vi "Output on.vi"(8 "error in (no error)":errorcluster, 10 "Output On":bool, 11 "Power Supply in":refnum<class "Power Supply.lvclass">) -> (0 "error out":errorcluster, 3 "Power Supply out":refnum<class "Power Supply.lvclass">)   [LabVIEW 2020, in "Power Supply.lvclass"]
uses:
  Power Supply.lvclass
  Power Supply.lvclass/Power Supply.ctl
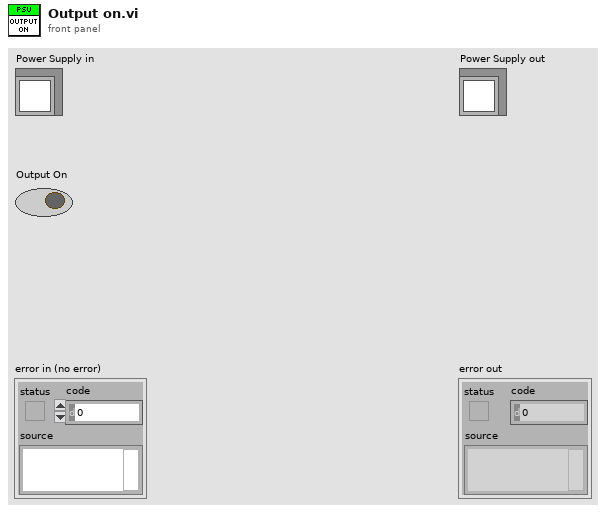
[diagram p1: front panel]
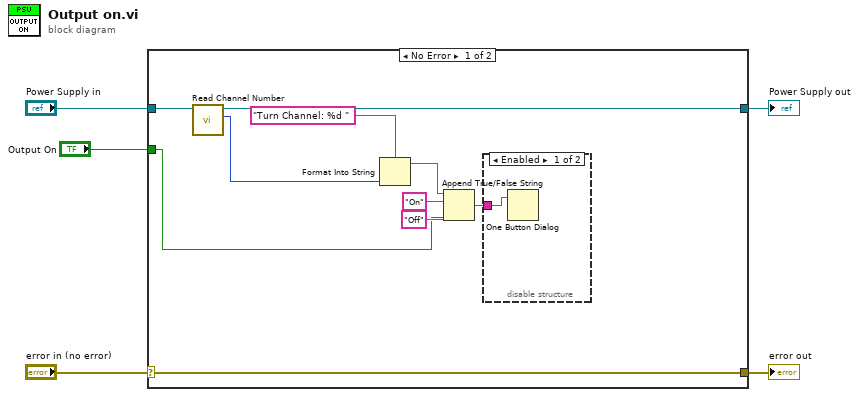
[diagram p0: block diagram]
diagram:
  n1 = case shown="No Error" "error in (no error)" {
    selector: "error in (no error)" -> [w15 w18]
    tunnel: [w15 w18] -> w4
    tunnel: [w7 w17] -> w2
    tunnel: "Power Supply in" -> [w8 w17]
    tunnel: "Output On" -> [w10 _]
    frame No Error {
      n2 = call "Read Channel Number.vi"("Power Supply in"=w8) -> ("Channel Number"=w6:u8, "Power Supply out"=w7:refnum<class "Power Supply.lvclass">)  [unwired: 9 in]
      n3 = Format Into String(format string="Turn Channel: %d ", w6) -> (resulting string=w13:string)  [unwired: 2 in, 1 out]
      n4 = Append True/False String(1:w10, 2:"Off" ("false string"), 3:"On" ("true string"), 4:w13) -> (0:w9:string)
      n5 = disable-structure shown="Enabled" {
        disable-tunnel: w9 -> [w16 _]
        frame Enabled {
          n6 = One Button Dialog(message=w16) -> ()  [unwired: 1 in, 1 out]
        }
        frame Disabled {
        }
      }
    }
    frame Error {
    }
  }
  "error out" <- w4
  "Power Supply out" <- w2
